vi "Release Session.vi"(0 "Session Handle":T1, 11 "error in (no error)":errorcluster, 13 "force destroy? (F)":bool) -> (15 "error out":errorcluster)   [LabVIEW 2020, in "HTS.lvlib" / "Execution.lvclass"]
doc: "Releases an obtained reference to the session"
uses:
  Execution.lvclass
  Typedefs/Session Handle.ctl
  C:/Program Files (x86)/National Instruments/LabVIEW 2020/user.lib/_Session Fwk/Session - Root.lvclass
  <userlib>/_Session Fwk/Session - Root.lvclass
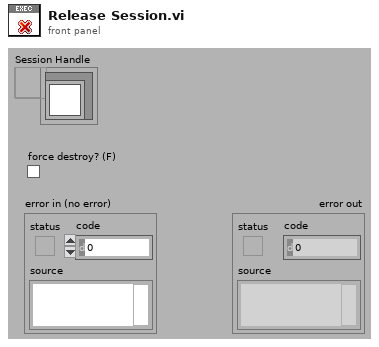
[diagram p1: front panel]
types:
  T1 = typedef "HTS.lvlib/Execution.lvclass/Session Handle.ctl" = refnum<data-value>
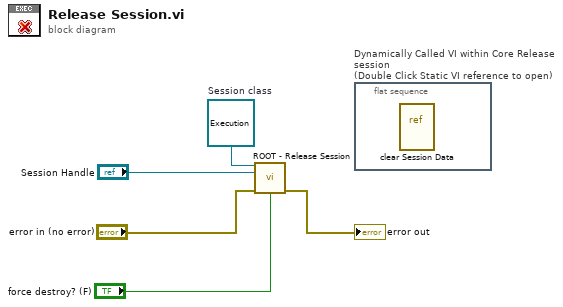
[diagram p0: block diagram]
diagram:
  w1 = refnum<class "Execution.lvclass"> refnum  # Session class
  n1 = call <userlib>:"ROOT - Release Session.vi"("OBJ - Session in"=w1, "Session Handle in"="Session Handle", "error in (no error)"="error in (no error)", "force destroy? (F)"="force destroy? (F)") -> ("error out"=→"error out":errorcluster)  [unwired: 10 in, 1 out]
  n2 = flat-sequence "Dynamically Called VI within Core Release session\n(Double Click Static VI reference to open)" {
    frame #0 {
      n3 = vi-ref "clear Session Data.vi"() -> ()  [unwired: 1 out]
    }
  }
